vi "RstEncoderCnt.vi"(8 "错误输入（无错误）":errorcluster) -> (0 "错误输出":errorcluster)   [LabVIEW 2014]
uses:
  X86Dll/ZXUTConfigMgr.dll
panel:
  in  "编码器端口号0~3":u8
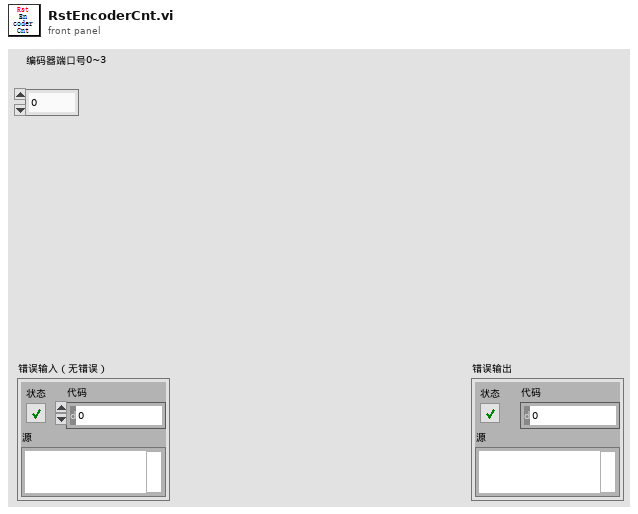
[diagram p1: front panel]
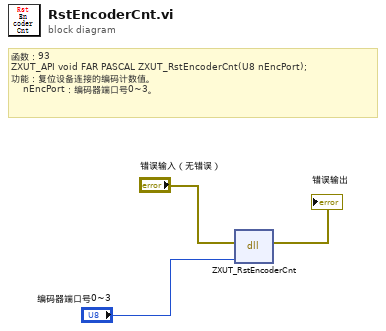
[diagram p0: block diagram]
diagram:
  # "函数：93\nZXUT_API void FAR PASCAL ZXUT_RstEncoderCnt(U8 nEncPort);\n功能：复位设备连接的编码计数值。\n\t   nEncPort：编码器端口号0~3。"
  n1 = dll-call lib="D:/Software/Utrasonic on-line monitoring/X86Dll/ZXUTConfigMgr.dll" fn="ZXUT_RstEncoderCnt"(error in="错误输入（无错误）", "nEncPort"="编码器端口号0~3") -> (error out=→"错误输出":errorcluster)  [unwired: 4 in, 1 out]
